vi "Circular_trajectory_of_tip_with_time.vi"() -> ()   [LabVIEW 2019]
uses:
  <vilib>/FPGAPlugInAG/sbRIO-9629/niLvFpga_Open_sbRIO-9629.vi
  <vilib>/rvi/interface/common/dynamic/niFpgaDynamicAddResources.vi
  <vilib>/Utility/error.llb/Error Cluster From Error Code.vi
  <vilib>/rvi/errors/niLvFpgaAdjustHostInterfaceError.vi
  <vilib>/FPGAPlugInAG/Dynamic/niLvFpga_Close_Dynamic.vi
  <vilib>/rvi/interface/nirviOpenFPGA/nirviOpenFPGA.xnode
  FPGA Bitfiles/fcmsinglesection_FPGATarget_ptuneof3motor_dYrR9swbniU.lvbitx
  Downloads/p tune of 3 motor.vi
  <vilib>/rvi/interface/nirviReadWriteControl/nirviReadWriteControl.xnode
  <vilib>/rvi/interface/nirviCloseFPGA/nirviCloseFPGA.xnode
  NiFpgaLv.dll
  <vilib>/rvi/interface/Simulation/niFpgaSimulationCallBeginRW.vi
panel:
  in  "Kp":dbl[](array[numeric])
  out "Error":dbl[](array[numeric])
  out "alpha 2":dbl
  out "L_v 2":dbl
  out "theta3 2":dbl
  out "theta2 2":dbl
  out "theta1 2":dbl
  out "Tip Position 2":dbl[](array[numeric])
  out "Marker ID":dbl
  out "Current Tip Coordinates(m)":dbl[](array[numeric])
  out "error out":errorcluster
  out "Z":dbl
  out "X":dbl
  out "Y":dbl
  out "Frame":dbl
  out "data out":string
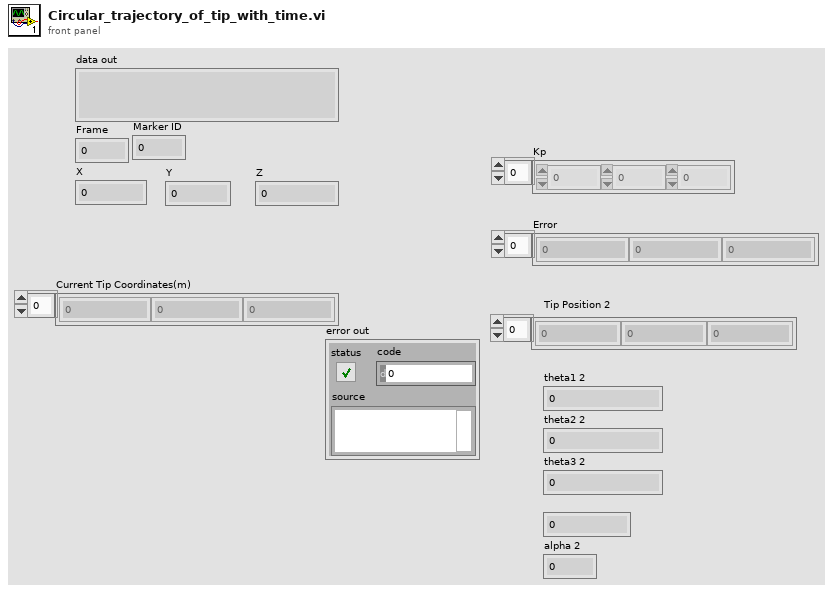
[diagram p1: front panel]
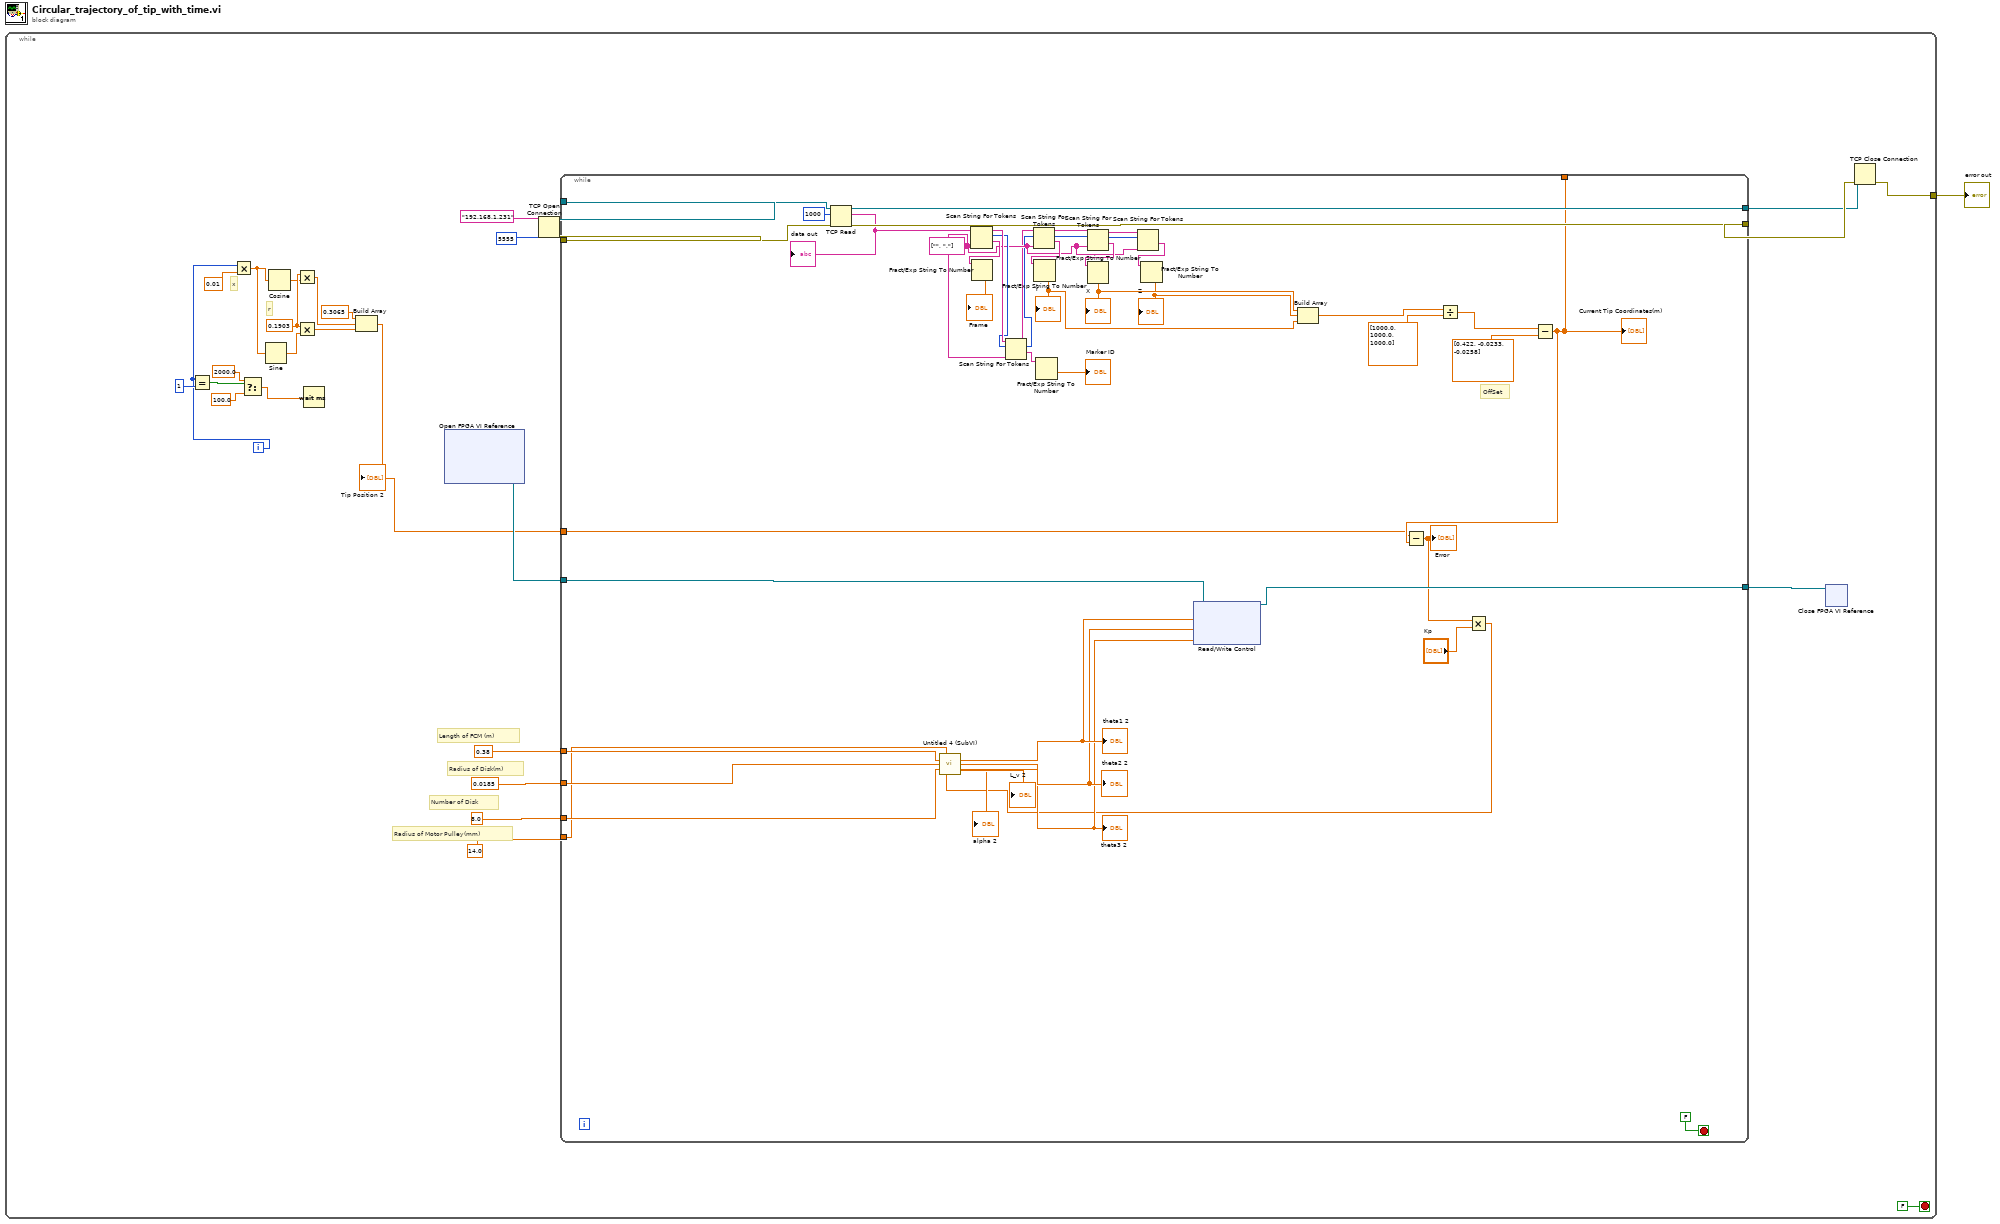
[diagram p0: block diagram]
diagram:
  n1 = while {
    tunnel: [w24] -> w1
    i -> [w7]
    stop <- FALSE stop-if-true
    w10 = 0.1903
    # "x"
    # "r"
    # "Radius of Motor Pulley(mm)"
    # "Number of Disk"
    # "Radius of Disk(m)"
    # "Length of FCM (m)"
    n2 = Equal?(x=w7, y=1) -> (x = y?=w17:bool)
    n3 = Multiply(x=w7, y=0.01) -> (x*y=w6:dbl)
    n4 = Select(t=2000.0, s=w17, f=100.0) -> (s? t:f=w16:dbl)
    n5 = Sine(x=w6) -> (sin(x)=w5:dbl)
    n6 = Cosine(x=w6) -> (cos(x)=w2:dbl)
    n7 = Multiply(x=w10, y=w2) -> (x*y=w3:dbl)
    n8 = Multiply(x=w10, y=w5) -> (x*y=w4:dbl)
    n9 = Wait (ms)(milliseconds to wait=w16) -> ()  [unwired: 1 out]
    n10 = Build Array(0.3065, w3, w4) -> (w9:dbl[])
    "Tip Position 2" <- w9
    n11 = xnode "Open FPGA VI Reference"() -> ("FPGA VI Reference Out"=w23:refnum<k20>)  [unwired: 2 in, 1 out]
    n12 = TCP Open Connection(address="192.168.1.231", remote port or service name=u16 5555) -> (connection ID=w29:refnum<k5>, error out=w30:errorcluster)  [unwired: 3 in]
    n13 = while {
      tunnel: [w75] -> w25
      tunnel: [w74] -> w26
      tunnel: w30 -> [w48]
      tunnel: w29 -> [w47]
      tunnel: [w33] -> _
      tunnel: w23 -> [w46]
      tunnel: [w45] -> w22
      tunnel: 8.0 ("Number of Disks") -> [w44]
      tunnel: 0.0185 ("Radius of disk (m)") -> [w43]
      tunnel: 0.38 ("Length of the FCM (m)") -> [w42]
      tunnel: 14.0 ("Radius of motor pulley\n (mm)") -> [w41]
      tunnel: w9 -> [w31]
      stop <- FALSE stop-if-true
      w51 = string[] ["", ","] ("delimiters (\\s,\\t,\\r,\\n)")
      # "OffSet"
      n14 = TCP Read(connection ID=w47, bytes to read=1000, error in (no error)=w48) -> (connection ID out=w75:refnum<k5>, data out=w72:string, error out=w74:errorcluster)  [unwired: 2 in]
      "data out" <- w72
      n15 = Scan String For Tokens(6:w51, 9:w72) -> (1:w67:string, 2:w54:i32, 3:w55:string)  [unwired: 4 in, 1 out]
      n16 = Fract/Exp String To Number(string=w67) -> (number=→"Frame":dbl)  [unwired: 3 in, 1 out]
      n17 = Scan String For Tokens(6:w51, 8:w54, 9:w55) -> (1:w53:string, 2:w49:i32, 3:w50:string)  [unwired: 3 in, 1 out]
      n18 = Scan String For Tokens(6:w51, 8:w49, 9:w50) -> (1:w66:string, 2:w69:i32, 3:w71:string)  [unwired: 3 in, 1 out]
      n19 = Fract/Exp String To Number(string=w66) -> (number=w56:dbl)  [unwired: 3 in, 1 out]
      "Y" <- w56
      n20 = Fract/Exp String To Number(string=w53) -> (number=→"Marker ID":dbl)  [unwired: 3 in, 1 out]
      n21 = Scan String For Tokens(6:w51, 8:w69, 9:w71) -> (1:w65:string, 2:w68:i32, 3:w70:string)  [unwired: 3 in, 1 out]
      n22 = Fract/Exp String To Number(string=w65) -> (number=w58:dbl)  [unwired: 3 in, 1 out]
      "X" <- w58
      n23 = Scan String For Tokens(6:w51, 8:w68, 9:w70) -> (1:w64:string)  [unwired: 3 in, 3 out]
      n24 = Fract/Exp String To Number(string=w64) -> (number=w57:dbl)  [unwired: 3 in, 1 out]
      "Z" <- w57
      n25 = Build Array(w58, w57, w56) -> (w62:dbl[])
      n26 = Divide(x=w62, y=dbl[] [1000.0, 1000.0, 1000.0]) -> (x/y=w60:dbl[])
      n27 = Subtract(x=w60, y=dbl[] [0.422, -0.0233, -0.0258]) -> (x-y=w33:dbl[])
      "Current Tip Coordinates(m)" <- w33
      n28 = Subtract(x=w31, y=w33) -> (x-y=w32:dbl[])
      "Error" <- w32
      n29 = Multiply(x=w32, y="Kp") -> (x*y=w34:dbl[])
      n30 = call "Untitled 4 (SubVI).vi"("Radius of motor pulley\n (mm)"=w41, "Length of the FCM (m)"=w42, "Radius of disk (m)"=w43, "Number of Disks"=w44, "Tip position Input"=w34) -> ("theta1"=w38:dbl, "theta2"=w37:dbl, "theta3"=w36:dbl, "L_v"=→"L_v 2":dbl, "alpha"=→"alpha 2":dbl)  [unwired: 2 in, 4 out]
      "theta1 2" <- w38
      "theta2 2" <- w37
      "theta3 2" <- w36
      n31 = xnode "Read/Write Control"("FPGA VI Reference In"=w46, "desired angle"=w38, "desired angle 2"=w37, "desired angle 3"=w36) -> ("FPGA VI Reference Out"=w45:refnum<k20>)  [unwired: 1 in, 1 out]
    }
    n32 = xnode "Close FPGA VI Reference"("FPGA VI Reference In"=w22) -> ()  [unwired: 1 in, 1 out]
    n33 = TCP Close Connection(connection ID=w25, error in (no error)=w26) -> (error out=w24:errorcluster)  [unwired: 1 in, 1 out]
  }
  "error out" <- w1
